vi "setUp.vi"(8 "error in (no error)":errorcluster, 11 "reference in":refnum<class "NI-SWITCH Import Export Unit Tests.lvclass">) -> (0 "error out":errorcluster, 3 "reference out":refnum<class "NI-SWITCH Import Export Unit Tests.lvclass">)   [LabVIEW 2017, in "NI-SWITCH Import Export Unit Tests.lvclass"]
doc: "setUp runs prior to the test method during test execution. Use this method to initialize any object data required by your tests."
uses:
  NI-SWITCH Import Export Unit Tests.lvclass
  C:/Program Files (x86)/National Instruments/LabVIEW 2017/vi.lib/addons/_JKI Toolkits/VI Tester/TestCase.llb/TestCase.lvclass
  NationalInstruments.VeriStand.SystemDefinitionAPI
  NI-SWITCH Import Export Unit Tests.lvclass/NI-SWITCH Import Export Unit Tests.ctl
  <userlib>/_OpenG.lib/file/file.llb/Append Path to Root if Relative - Scalar__ogtk.vi
  <vilib>/addons/_JKI Toolkits/VI Tester/TestCase.llb/TestCase.lvclass
  niveristand-custom-device-testing-tools/VeriStandTestUtilities/VeriStandTestUtilities.lvlib
  Shared/VeriStand SLSC Scripting/VeriStand SLSC Scripting.lvlib
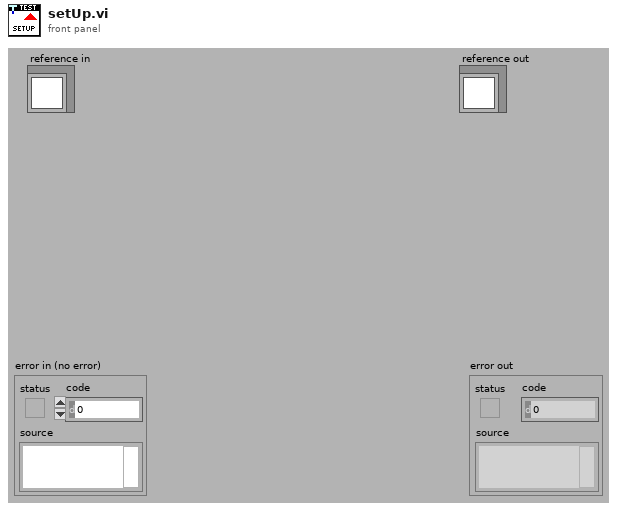
[diagram p1: front panel]
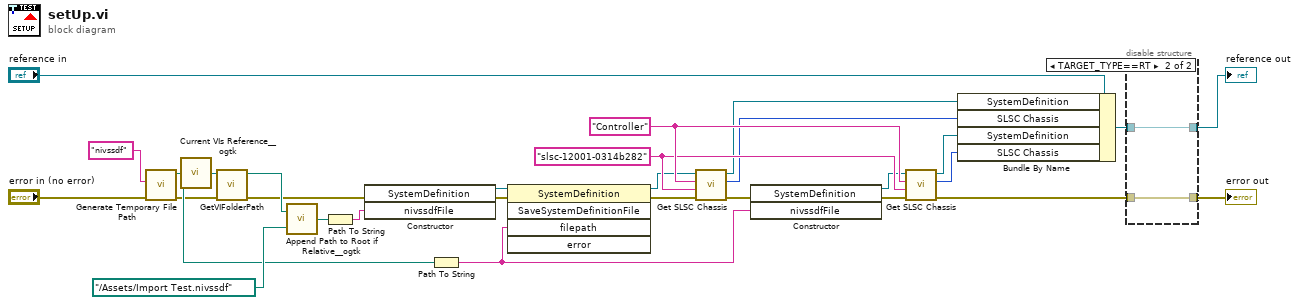
[diagram p0: block diagram]
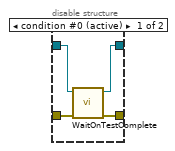
[diagram p2: hidden frame]
diagram:
  w11 = "slsc-12001-0314b282" ("Name or IP")
  w12 = "Controller" ("Target")
  n1 = call <vilib>:"Generate Temporary File Path.vi"("error in (no error)"="error in (no error)", "Temporary File Extension (tmp)"="nivssdf") -> ("error out"=w2:errorcluster, "Unique Temporary File Path"=w18:path)  [unwired: 8 in]
  n2 = call <userlib>:"Current VIs Reference__ogtk.vi"() -> ("Current VI's reference"=w27:refnum<vi>)  [unwired: 5 in]
  n3 = call "GetVIFolderPath.vi"("error in (no error)"=w2, "VI Reference in"=w27) -> ("error out"=w3:errorcluster, "VI Folder Path out"=w26:path)  [unwired: 8 in]
  n4 = call-poly <userlib>:"Append Path to Root if Relative__ogtk.vi"("Absolute or Relative Path"=path "../Assets/Import Test.nivssdf", "Root Path"=w26) -> ("Absolute or Appended Path"=w24:path)
  n5 = Path To String(path=w24) -> (string=w23:string)
  n6 = constructor class="SystemDefinition"(error in=w3, "nivssdfFile"=w23) -> (reference out=w17:refnum<k24>, error out=w4:errorcluster)  [unwired: 2 in, 2 out]
  n7 = Path To String(path=w18) -> (string=w16:string)
  n8 = invoke class="SystemDefinition" method="SaveSystemDefinitionFile"(reference=w17, error in=w4, "filepath"=w16) -> (reference out=w10:refnum<k24>, error out=w14:errorcluster)  [unwired: 2 in, 3 out]
  n9 = call "Get SLSC Chassis.vi"("error in (no error)"=w14, "SLSC Chassis Name or IP"=w11, "Target Name"=w12, "SysDef in"=w10) -> ("error out"=w13:errorcluster, "SLSC Chassis"=w6:u64, "SysDef out"=w5:refnum<k24>)  [unwired: 4 in, 1 out]
  n10 = constructor class="SystemDefinition"(error in=w13, "nivssdfFile"=w16) -> (reference out=w9:refnum<k24>, error out=w15:errorcluster)  [unwired: 2 in, 2 out]
  n11 = call "Get SLSC Chassis.vi"("error in (no error)"=w15, "SLSC Chassis Name or IP"=w11, "Target Name"=w12, "SysDef in"=w9) -> ("error out"=w22:errorcluster, "SLSC Chassis"=w8:u64, "SysDef out"=w7:refnum<k24>)  [unwired: 4 in, 1 out]
  n12 = Bundle By Name(cluster="reference in", "SystemDefinition"=w5, "SLSC Chassis"=w6, "SystemDefinition"=w7, "SLSC Chassis"=w8) -> (w20:refnum<class "NI-SWITCH Import Export Unit Tests.lvclass">)
  n13 = disable-structure shown="TARGET_TYPE==RT" {
    disable-tunnel: w22 -> [w33 w34]
    disable-tunnel: [w32 w34] -> w29
    disable-tunnel: [w31 w35] -> w28
    disable-tunnel: w20 -> [w30 w35]
    frame condition #0 (active) {
      n14 = call <vilib>:"WaitOnTestComplete.vi"("error in (no error)"=w33, "TestCase in"=w30) -> ("error out"=w32:errorcluster, "TestCase out"=w31:refnum<class "NI-SWITCH Import Export Unit Tests.lvclass">)  [unwired: 8 in]
    }
    frame condition #1 {
    }
  }
  "error out" <- w29
  "reference out" <- w28
